vi "自我介绍.vi"(8 "error in (no error)":errorcluster caption="错误输入（无错误）", 11 "鸭子库.lvlib:红头鸭.lvclass":refnum<class "红头鸭.lvclass">) -> (0 "error out":errorcluster caption="错误输出", 3 "鸭子库.lvlib:红头鸭.lvclass":refnum<class "红头鸭.lvclass">)   [LabVIEW 2022 SP3, in "鸭子库.lvlib" / "红头鸭.lvclass"]
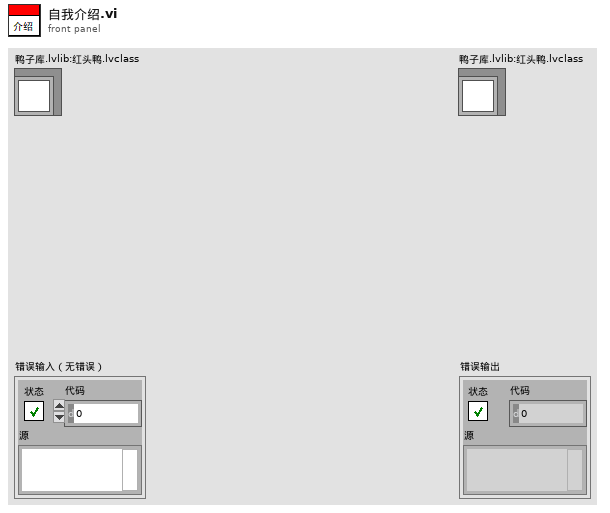
[diagram p1: front panel]
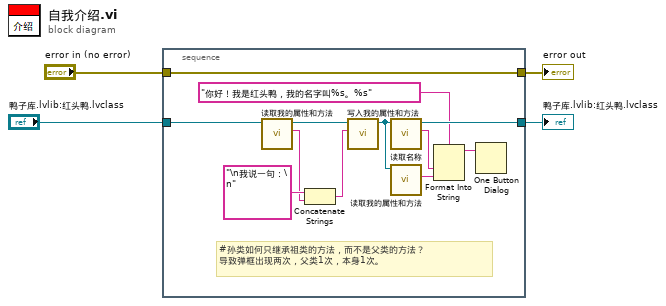
[diagram p0: block diagram]
diagram:
  n1 = stacked-sequence {
    tunnel: [w11] -> w4
    tunnel: [w16] -> w3
    tunnel: "error in (no error)" -> [w11]
    tunnel: "鸭子库.lvlib:红头鸭.lvclass" -> [w6]
    frame #0 {
      # "#孙类如何只继承祖类的方法，而不是父类的方法？\n导致弹框出现两次，父类1次，本身1次。"
      n2 = call "读取我的属性和方法.vi"("鸭子输入"=w6) -> ("我的属性和方法"=w8:string, "鸭子输出"=w7:refnum<class "红头鸭.lvclass">)  [unwired: 8 in, 1 out]
      n3 = Concatenate Strings("\n我说一句：\n" ("字符串"), w8) -> (w10:string)
      n4 = call "写入我的属性和方法.vi"("我的属性和方法"=w10, "鸭子输入"=w7) -> ("鸭子输出"=w5:refnum<class "红头鸭.lvclass">)  [unwired: 8 in, 1 out]
      n5 = call "读取名称.vi"("鸭子库.lvlib:鸭子.lvclass"=w5) -> ("名称"=w15:string, "鸭子库.lvlib:鸭子.lvclass"=w16:refnum<class "红头鸭.lvclass">)  [unwired: 8 in, 1 out]
      n6 = call "读取我的属性和方法.vi"("鸭子输入"=w5) -> ("我的属性和方法"=w14:string)  [unwired: 8 in, 2 out]
      n7 = Format Into String(format string="你好！我是红头鸭，我的名字叫%s。%s" ("格式字符串"), w15, w14) -> (resulting string=w13:string)  [unwired: 2 in, 1 out]
      n8 = One Button Dialog(message=w13) -> ()  [unwired: 1 in, 1 out]
    }
  }
  "error out" <- w4
  "鸭子库.lvlib:红头鸭.lvclass" <- w3
